vi "Select filepath if none.vi"(2 "Error message":string="Must select a file." caption="Message", 3 "Selector prompt":string="Select a file", 4 "Filepath in":path) -> (0 "Filepath valid?":bool, 1 "Filepath out":path)   [LabVIEW 2015]
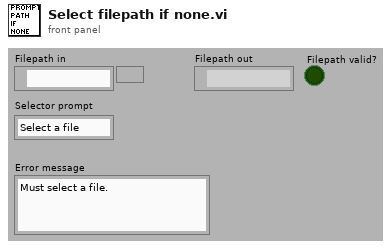
[diagram p1: front panel]
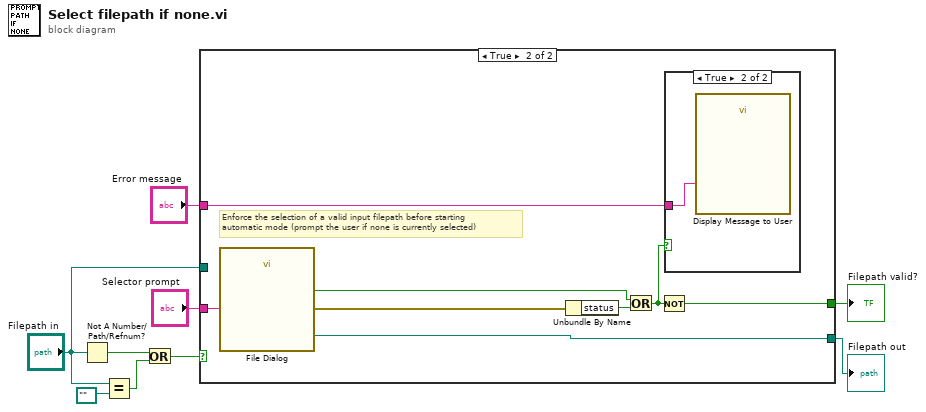
[diagram p0: block diagram]
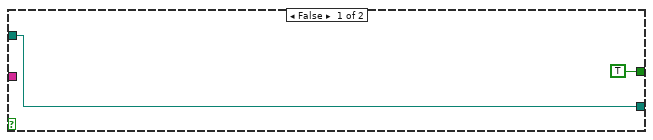
[diagram p2: hidden frame]
diagram:
  n1 = Not A Number/Path/Refnum?(number/path/refnum="Filepath in") -> (NaN/Path/Refnum?=w5:bool)
  n2 = Equal?(x="Filepath in", y=path "") -> (x = y?=w4:bool)
  n3 = Or(x=w5, y=w4) -> (x .or. y?=w9:bool)
  n4 = case shown="True" w9 {
    tunnel: "Filepath in" -> [w11 _]
    tunnel: [w11 w16] -> w7
    tunnel: [TRUE w14] -> w8
    tunnel: "Error message" -> [_ w13]
    tunnel: "Selector prompt" -> [_ w12]
    frame False {
    }
    frame True {
      # "Enforce the selection of a valid input filepath before starting\nautomatic mode (prompt the user if none is currently selected)"
      n5 = call "File Dialog"("prompt"=w12) -> ("selected path"=w16:path, "cancelled"=w17:bool, "error out"=w19:errorcluster)  [unwired: 11 in, 1 out]
      n6 = Unbundle By Name(w19) -> ("status"=w18:bool)
      n7 = Or(x=w17, y=w18) -> (x .or. y?=w15:bool)
      n8 = Not(x=w15) -> (.not. x?=w14:bool)
      n9 = case shown="True" w15 {
        tunnel: w13 -> [_ w20]
        frame False {
        }
        frame True {
          n10 = call "Display Message to User"("Message"=w20) -> ()  [unwired: 9 in, 2 out]
        }
      }
    }
  }
  "Filepath valid?" <- w8
  "Filepath out" <- w7
